vi "Teleop.vi"(10 "Match Info":T1={"Autonomous Elapsed Seconds"=0.0, "TeleOp Elapsed Seconds"=0.0, "Disabled Elapsed Seconds"=0.0, "Visited Autonomous"=FALSE, "Visited TeleOp"=FALSE, "Visited Disabled"=FALSE, "Autonomous Settings"={"Autonomous Style"=enum."Independent", "VI Refnum"=refnum}}, 11 "Call Context":T2) -> ()   [LabVIEW 2018]
doc: "This VI is called for each TeleOp packet received from the DS where the robot is not disabled. It is often used to read from the joysticks and update I/O or to update setpoints for timed control loops. It should complete and return within 20 milliseconds or it may miss DS packets."
uses:
  <vilib>/Rock Robotics/WPI/DriverStation/WPI_DriverStationDerivedRobotMode.ctl
  <vilib>/Rock Robotics/WPI/DriverStation/WPI_DriverStationMatch Info.ctl
  <vilib>/Rock Robotics/WPI/ThirdParty/Phoenix-LabVIEW/Motor Controller/Controls/CTRE_Phoenix_MotorControl_ControlMode.ctl
  <vilib>/Rock Robotics/WPI/Solenoid/WPI_SolenoidValue.ctl
  <vilib>/Rock Robotics/Network Tables/NT Read Boolean.vi
  <vilib>/Rock Robotics/Network Tables/NT Read Number.vi
  <vilib>/Rock Robotics/WPI/Utilities/WPI_GetSetVariantRefNum.vi
  <vilib>/Rock Robotics/WPI/Solenoid/WPI_SolenoidSetEnum.vi
  <vilib>/Rock Robotics/WPI/ThirdParty/Phoenix-LabVIEW/Motor Controller/Get/CTRE_Phoenix_MotorController_GetSelectedSensorData.vi
  <vilib>/Rock Robotics/WPI/RobotDrive/WPI_RobotDriveArcadeDrive_Standard(NoSaturation).vi
panel:
  out "Sample Slider 0":dbl(slide) scale=0.0..5.0
  out "Sample Boolean 1":bool
  out "Sample Boolean 0":bool
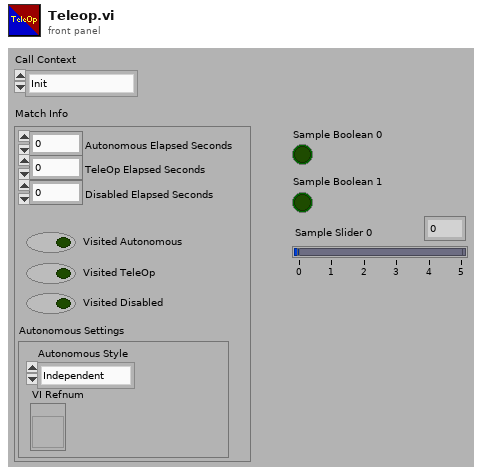
[diagram p1: front panel]
types:
  T1 = typedef "WPI_DriverStationMatch Info.ctl" = cluster{"Autonomous Elapsed Seconds":dbl, "TeleOp Elapsed Seconds":dbl, "Disabled Elapsed Seconds":dbl, "Visited Autonomous":bool, "Visited TeleOp":bool, "Visited Disabled":bool, "Autonomous Settings":cluster{"Autonomous Style":enum16{"Iterative", "Independent"}, "VI Refnum":refnum<vi>}}
  T2 = typedef "WPI_DriverStationDerivedRobotMode.ctl" = enum16{"Init", "Execute", "Stop"}
  T3 = typedef "WPI_MotorControlDeviceRef.ctl" = cluster{"DeviceStatus":errorcluster, "Type":T4, "PWM":cluster{"PWM Channel":T5, "DeadBand":T6}, "CAN":cluster{"Device Number":u8, "SetOutput VI Ref":variant, "GetOutput VI Ref":variant, "Enable VI Ref":variant, "Disable VI Ref":variant, "Data":variant}, "Invert":bool, "DIO PWM":cluster{"PWM \"Enable\" Channel":T5, "DIOChannel":T7, "PWM Rate":dbl}}
  T4 = typedef "WPI_MotorControlType.ctl" = enum16{"PWM", "CAN", "DIO PWM"}
  T5 = typedef "FPGA_DIOPWMChannel.ctl" = enum8{"PWM 0", "PWM 1", "PWM 2", "PWM 3", "PWM 4", "PWM 5", "PWM 6", "PWM 7", "PWM 8", "PWM 9", "PWM MXP 0", "PWM MXP 1", "PWM MXP 2", "PWM MXP 3", "PWM MXP 4", "PWM MXP 5", "PWM MXP 6", "PWM MXP 7", "PWM MXP 8", "PWM MXP 9", "Invalid"}
  T6 = typedef "WPI_PWMDeadband.ctl" = cluster{"Name":string, "maxPositivePwm":i32, "minPositivePwm":i32, "centerPwm":i32, "maxNegativePwm":i32, "minNegativePwm":i32, "angularRange":u16}
  T7 = typedef "FPGA_DIOChannel.ctl" = enum8{"DIO 0", "DIO 1", "DIO 2", "DIO 3", "DIO 4", "DIO 5", "DIO 6", "DIO 7", "DIO 8", "DIO 9", "DIO MXP 0", "DIO MXP 1", "DIO MXP 2", "DIO MXP 3", "DIO MXP 4", "DIO MXP 5", "DIO MXP 6", "DIO MXP 7", "DIO MXP 8", "DIO MXP 9", "DIO MXP 10", "DIO MXP 11", "DIO MXP 12", "DIO MXP 13", "DIO MXP 14", "DIO MXP 15", "SPI Port CS1", "SPI Port CS2", "SPI Port CS3", "SPI Port MISO", "SPI Port MOSI", "Invalid"}
  T8 = typedef "CTRE_Phoenix_MotorControl_ControlMode.ctl" = u16
  T9 = typedef "WPI_SolenoidDevRef.ctl" = cluster{"DevStatus":errorcluster, "Pneumatics Control Module":u8, "Forward Solenoid Channel":T10, "Reverse Solenoid Channel":T10}
  T10 = typedef "WPI_SolenoidChannel.ctl" = enum8{"Solenoid 0", "Solenoid 1", "Solenoid 2", "Solenoid 3", "Solenoid 4", "Solenoid 5", "Solenoid 6", "Solenoid 7", "Invalid"}
  T11 = typedef "WPI_SolenoidValue.ctl" = enum16{"Off", "On", "Forward", "Reverse"}
  T12 = typedef "WPI_RobotDriveDevRef.ctl" = cluster{"DevStatus":errorcluster, "Motors[]":T3[], "Square Inputs":bool, "Max Output":dbl}
  T13 = typedef "WPI_JoystickDevRef.ctl" = cluster{"Device":T14}
  T14 = typedef "WPI_JoystickDeviceEnum.ctl" = enum16{"USB 0", "USB 1", "USB 2", "USB 3", "USB 4", "USB 5"}
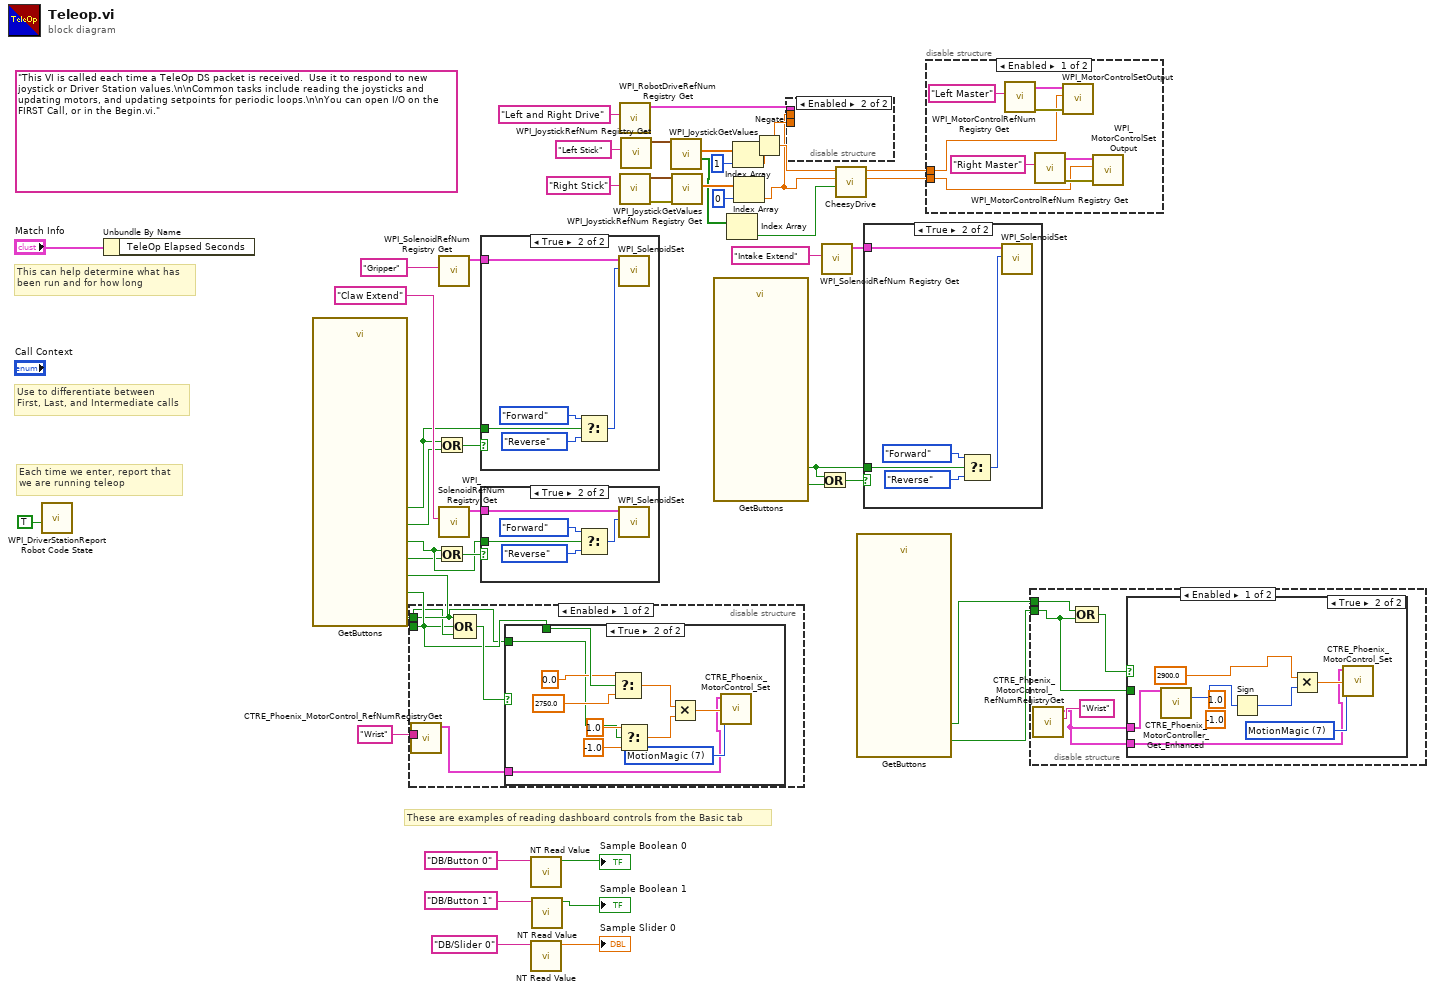
[diagram p0: block diagram]
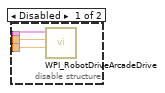
[diagram p5: hidden frame]
diagram:
  (unwired) "This VI is called each time a TeleOp DS packet is received.  Use it to respond to new joystick or Driver Station values.\n\nCommon tasks include reading the joysticks and updating motors, and updating setpoints for periodic loops.\n\nYou can open I/O on the FIRST Call, or in the Begin.vi."
  # "These are examples of reading dashboard controls from the Basic tab"
  # "Each time we enter, report that\nwe are running teleop"
  # "Use to differentiate between\nFirst, Last, and Intermediate calls"
  # "This can help determine what has\nbeen run and for how long"
  n1 = call <vilib>:"WPI_DriverStationReport Robot Code State.vi"("TeleOp"=TRUE ("Autonomous")) -> ()  [unwired: 10 in, 1 out]
  n2 = Unbundle By Name("Match Info") -> ()  [unwired: 1 out]
  n3 = call "GetButtons.vi"() -> ("Claw Open"=w36:bool, "Claw Close"=w35:bool, "Rollers In"=w32:bool, "Rollers Out"=w33:bool, "Wrist Out"=w26:bool, "Wrist Stow"=w28:bool, "Wrist Score"=w27:bool)  [unwired: 13 out]
  n4 = disable-structure shown="Enabled" {
    disable-tunnel: "Wrist" ("refnum name") -> [w53 _]
    disable-tunnel: w28 -> [w52 _]
    disable-tunnel: w27 -> [w50 _]
    disable-tunnel: w26 -> [w49 _]
    frame Enabled {
      n5 = call <vilib>:"CTRE_Phoenix_MotorControl_RefNumRegistryGet.vi"("refnum name"=w53) -> ("PhoenixMotorControlDevRef"=w48:T3)  [unwired: 9 in, 1 out]
      n6 = Compound Arithmetic op=OR(w49, w50, w52) -> (w51:bool)
      n7 = case shown="True" w51 {
        tunnel: w50 -> [_ w64]
        tunnel: w49 -> [_ w57]
        tunnel: w48 -> [_ w54]
        frame False {
        }
        frame True {
          w55 = T8 7 items=["PercentOutput"=0, "Position"=1, "Velocity"=2, "Current"=3, "Follower"=5, "MotionProfile"=6, "MotionMagic"=7, "MotionProfileArc"=10, "Disabled"=15] ("Control Mode")
          n8 = Select(t=0.0, s=w64, f=2750.0 ("t")) -> (s? t:f=w63:dbl)
          n9 = Select(t=1.0, s=w57, f=-1.0) -> (s? t:f=w62:dbl)
          n10 = Multiply(x=w63, y=w62) -> (x*y=w56:dbl)
          n11 = call <vilib>:"CTRE_Phoenix_MotorControl_Set.vi"("Output"=w56, "Control Mode"=w55, "PhoenixMotorControlDevRef"=w54) -> ()  [unwired: 7 in, 2 out]
        }
      }
    }
    frame Disabled {
    }
  }
  n12 = Or(x=w36, y=w35) -> (x .or. y?=w37:bool)
  n13 = Or(x=w33, y=w32) -> (x .or. y?=w34:bool)
  n14 = call <vilib>:"WPI_SolenoidRefNum Registry Get.vi"("refnum name"="Gripper") -> ("SolenoidDevRef"=w30:T9)  [unwired: 9 in, 1 out]
  n15 = call <vilib>:"WPI_SolenoidRefNum Registry Get.vi"("refnum name"="Claw Extend") -> ("SolenoidDevRef"=w31:T9)  [unwired: 9 in, 1 out]
  n16 = case shown="True" w37 {
    tunnel: w36 -> [_ w69]
    tunnel: w30 -> [_ w65]
    frame False {
    }
    frame True {
      n17 = Select(t=WPI_SolenoidValue."Forward" ("Value"), s=w69, f=WPI_SolenoidValue."Reverse" ("Value")) -> (s? t:f=w66:T11)
      n18 = call-poly <vilib>:"WPI_SolenoidSet.vi"("Value"=w66, "SolenoidDevRef"=w65) -> ()  [unwired: 8 in, 2 out]
    }
  }
  n19 = case shown="True" w34 {
    tunnel: w33 -> [_ w74]
    tunnel: w31 -> [_ w70]
    frame False {
    }
    frame True {
      n20 = Select(t=WPI_SolenoidValue."Forward" ("Value"), s=w74, f=WPI_SolenoidValue."Reverse" ("Value")) -> (s? t:f=w71:T11)
      n21 = call-poly <vilib>:"WPI_SolenoidSet.vi"("Value"=w71, "SolenoidDevRef"=w70) -> ()  [unwired: 8 in, 2 out]
    }
  }
  n22 = call-poly <vilib>:"NT Read Value.vi"("Name"="DB/Button 0" ("refnum name")) -> ("Boolean"=→"Sample Boolean 0":bool)  [unwired: 9 in, 1 out]
  n23 = call-poly <vilib>:"NT Read Value.vi"("Name"="DB/Slider 0" ("refnum name")) -> ("Numeric"=→"Sample Slider 0":dbl)  [unwired: 9 in, 1 out]
  n24 = call-poly <vilib>:"NT Read Value.vi"("Name"="DB/Button 1" ("refnum name")) -> ("Boolean"=→"Sample Boolean 1":bool)  [unwired: 9 in, 1 out]
  n25 = call <vilib>:"WPI_RobotDriveRefNum Registry Get.vi"("refnum name"="Left and Right Drive") -> ("RobotDriveDevRef"=w22:T12)  [unwired: 9 in, 1 out]
  n26 = call <vilib>:"WPI_JoystickRefNum Registry Get.vi"("refnum name"="Right Stick") -> ("error out"=w18:errorcluster, "JoystickDevRef"=w17:T13)  [unwired: 9 in]
  n27 = call <vilib>:"WPI_JoystickRefNum Registry Get.vi"("refnum name"="Left Stick") -> ("JoystickDevRef"=w21:T13)  [unwired: 9 in, 1 out]
  n28 = call <vilib>:"WPI_JoystickGetValues.vi"("JoystickDevRef"=w21) -> ("Buttons"=w7:bool[], "Axes"=w20:dbl[])  [unwired: 6 in, 3 out]
  n29 = call <vilib>:"WPI_JoystickGetValues.vi"("error in (no error)"=w18, "JoystickDevRef"=w17) -> ("Axes"=w19:dbl[])  [unwired: 5 in, 4 out]
  n30 = call "GetButtons.vi"() -> ("Exchange In"=w9:bool, "Exchange Out"=w10:bool)  [unwired: 18 out]
  n31 = Index Array(array=w7) -> (element=w6:bool)  [unwired: 1 in]
  n32 = Index Array(array=w20, index=1) -> (element=w14:dbl)
  n33 = Index Array(array=w19, index=0) -> (element=w1:dbl)
  n34 = Negate(x=w14) -> (-x=w8:dbl)
  n35 = disable-structure shown="Enabled" {
    disable-tunnel: w22 -> [w77 _]
    disable-tunnel: w8 -> [w76 _]
    disable-tunnel: w1 -> [w75 _]
    frame Disabled {
      n36 = call-poly <vilib>:"WPI_RobotDriveArcadeDrive.vi"("Y axis value"=w76, "X axis value"=w75, "RobotDriveDevRef"=w77) -> ()  [unwired: 6 in, 3 out]
    }
    frame Enabled {
    }
  }
  n37 = Or(x=w10, y=w9) -> (x .or. y?=w13:bool)
  n38 = call <vilib>:"WPI_SolenoidRefNum Registry Get.vi"("refnum name"="Intake Extend") -> ("SolenoidDevRef"=w12:T9)  [unwired: 9 in, 1 out]
  n39 = call "CheesyDrive.vi"("Quick Turn"=w6, "Turn"=w1, "Throttle"=w8) -> ("Right Motor Value"=w5:dbl, "Left Motor Value"=w4:dbl)  [unwired: 7 in]
  n40 = call "GetButtons.vi"() -> ("Switch"=w3:bool, "Switch 2"=w2:bool)  [unwired: 18 out]
  n41 = case shown="True" w13 {
    tunnel: w10 -> [_ w82]
    tunnel: w12 -> [_ w78]
    frame False {
    }
    frame True {
      n42 = Select(t=WPI_SolenoidValue."Forward" ("Value"), s=w82, f=WPI_SolenoidValue."Reverse" ("Value")) -> (s? t:f=w79:T11)
      n43 = call-poly <vilib>:"WPI_SolenoidSet.vi"("Value"=w79, "SolenoidDevRef"=w78) -> ()  [unwired: 8 in, 2 out]
    }
  }
  n44 = disable-structure shown="Enabled" {
    disable-tunnel: w5 -> [w84 _]
    disable-tunnel: w4 -> [w83 _]
    frame Enabled {
      n45 = call <vilib>:"WPI_MotorControlRefNum Registry Get.vi"("refnum name"="Left Master") -> ("error out"=w89:errorcluster, "MotorControlDevRef"=w90:T3)  [unwired: 9 in]
      n46 = call <vilib>:"WPI_MotorControlRefNum Registry Get.vi"("refnum name"="Right Master") -> ("error out"=w86:errorcluster, "MotorControlDevRef"=w87:T3)  [unwired: 9 in]
      n47 = call <vilib>:"WPI_MotorControlSetOutput.vi"("error in (no error)"=w89, "Output"=w83, "MotorControlDevRef"=w90) -> ()  [unwired: 6 in, 3 out]
      n48 = call <vilib>:"WPI_MotorControlSetOutput.vi"("error in (no error)"=w86, "Output"=w84, "MotorControlDevRef"=w87) -> ()  [unwired: 6 in, 3 out]
    }
    frame Disabled {
    }
  }
  n49 = disable-structure shown="Enabled" {
    disable-tunnel: w3 -> [w94 _]
    disable-tunnel: w2 -> [w93 _]
    frame Enabled {
      n50 = call <vilib>:"CTRE_Phoenix_MotorControl_RefNumRegistryGet.vi"("refnum name"="Wrist") -> ("PhoenixMotorControlDevRef"=w91:T3)  [unwired: 9 in, 1 out]
      n51 = Compound Arithmetic op=OR(w94, w93) -> (w95:bool)
      n52 = case shown="True" w95 {
        tunnel: w91 -> [_ w100]
        tunnel: w93 -> [_ _]
        tunnel: w91 -> [_ w96]
        frame False {
        }
        frame True {
          w101 = T8 7 items=["PercentOutput"=0, "Position"=1, "Velocity"=2, "Current"=3, "Follower"=5, "MotionProfile"=6, "MotionMagic"=7, "MotionProfileArc"=10, "Disabled"=15] ("Control Mode")
          (unwired) -1.0 ("f")
          (unwired) 1.0 ("t")
          n53 = call-poly <vilib>:"CTRE_Phoenix_MotorController_Get_Enhanced.vi"("PhoenixMotorControlDevRef"=w96) -> ("Position (Raw Sensor Units)"=w98:i32)  [unwired: 11 in, 3 out]
          n54 = Sign(1:w98) -> (0:w97:i32)
          n55 = Multiply(x=2900.0 ("t"), y=w97) -> (x*y=w102:dbl)
          n56 = call <vilib>:"CTRE_Phoenix_MotorControl_Set.vi"("Output"=w102, "Control Mode"=w101, "PhoenixMotorControlDevRef"=w100) -> ()  [unwired: 7 in, 2 out]
        }
      }
    }
    frame Disabled {
    }
  }
